vi "open.vi"(8 "error in (no error)":errorcluster caption="错误输入（无错误）", 11 "EPEVER-MPPT 输入":refnum<class "EPEVER-MPPT.lvclass">) -> (0 "error out":errorcluster caption="错误输出", 3 "EPEVER-MPPT 输出":refnum<class "EPEVER-MPPT.lvclass">)   [LabVIEW 2016, in "EPEVER-MPPT.lvlib" / "EPEVER-MPPT.lvclass"]
uses:
  EPEVER-MPPT.lvclass
  EPEVER-MPPT.lvclass/EPEVER-MPPT.ctl
  <vilib>/Plasmionique/MB Master/MB_Master_Serial/MB_Master_Serial.lvclass
  C:/Program Files (x86)/National Instruments/LabVIEW 2016/vi.lib/Plasmionique/MB Master/MB_Master/MB_Master.lvclass
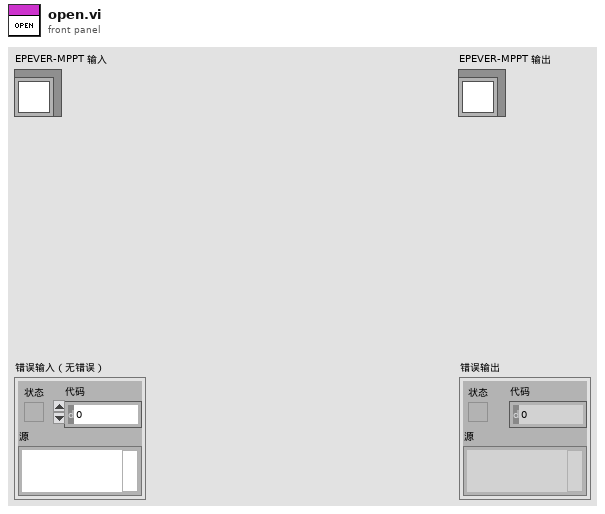
[diagram p1: front panel]
types:
  T1 = cluster{"baud rate (bps)":u32, "stop bits":u16, "parity":u16, "flow control":u16, "timeout":u32, "retries":i32}
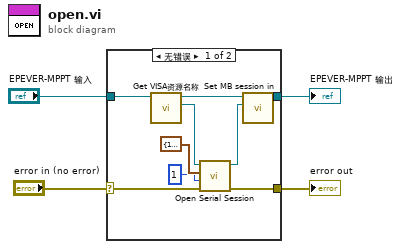
[diagram p0: block diagram]
diagram:
  n1 = case shown="无错误" "error in (no error)" {
    selector: "error in (no error)" -> [w6 w15]
    tunnel: [w5 w15] -> w3
    tunnel: [w7 w14] -> w1
    tunnel: "EPEVER-MPPT 输入" -> [w13 w14]
    frame No Error {
      n2 = call "Get VISA资源名称.vi"("EPEVER-MPPT in"=w13) -> ("VISA资源名称"=w12:refnum<visa-resource-name>, "EPEVER-MPPT out"=w10:refnum<class "EPEVER-MPPT.lvclass">)  [unwired: 9 in]
      n3 = call <vilib>:"Open Serial Session.vi"("Error in"=w6, "Slave ID"=u8 1, "Serial Config"=T1 {"baud rate (bps)"=115200, "stop bits"=10, "parity"=0, "flow control"=0, "timeout"=1000, "retries"=1}, "VISA Resource"=w12) -> ("Error out"=w5:errorcluster, "MB_Serial session"=w9:refnum<class "MB_Master_Serial.lvclass">)  [unwired: 6 in]
      n4 = call "Set MB session in.vi"("MB Serial Master:MB_Master"=w9, "EPEVER-MPPT in"=w10) -> ("EPEVER-MPPT out"=w7:refnum<class "EPEVER-MPPT.lvclass">)  [unwired: 9 in]
    }
    frame Error {
    }
  }
  "error out" <- w3
  "EPEVER-MPPT 输出" <- w1
